vi "poly test (string).vi"(1 "String":string) -> (0 "String out":string)   [LabVIEW 2012]
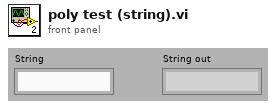
[diagram p1: front panel]
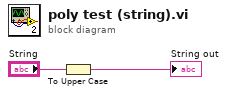
[diagram p0: block diagram]
diagram:
  n1 = To Upper Case(1:"String") -> (0:→"String out":string)
